vi "Read Field (Variant).vi"(7 "field name":string, 8 "error in (no error)":errorcluster, 9 "type code":T1, 10 "value":variant, 11 "PV Data in":refnum<class "PV Data.lvclass">) -> (0 "error out":errorcluster, 1 "type code out":T1, 2 "value out":variant, 3 "PV Data out":refnum<class "PV Data.lvclass">)   [LabVIEW 2020, in "PV Access.lvlib" / "PV Data.lvlib" / "PV Data.lvclass"]
uses:
  PV Data.lvclass
  PV Data.lvclass/PV Data.ctl
  <vilib>/ErrorRing/Error Ring.xnode
  3e63842f-1b42-44b7-bfbc-53574ae558bd.vi
  0df52538-0c37-4fc1-a2a6-aa64d23bd73e.vi
  ea7cb730-9445-4e63-a674-7488b051f0a2.vi
  ecc6d044-d1d6-4258-b554-93b542f000c4.vi
  f0dd0353-13dc-4229-be36-72f5216b3ba3.vi
  663b7534-5be4-4c26-8693-775dffd107bf.vi
  6d95b702-a3d4-47fa-b99c-6e9c691d9abd.vi
  334379f0-c2c1-4fd4-b37a-a75153a3c3c1.vi
  22215a59-2fe5-468e-8a76-07a567f1422d.vi
  3b673ad6-c2bb-415d-ac32-dac8d0585a62.vi
  4907590c-51dd-452d-854a-3f23d6337043.vi
  91e94b60-106e-4a8f-bb72-5d9817169e6a.vi
  c7390ac7-e1e0-4f30-b90a-9159575d946d.vi
  aaf6655d-cd8e-45f8-b77e-a22837ed21e0.vi
  830d96f2-0dcb-4e12-99cb-9e6dde05f73e.vi
  77dc8c9c-6059-4e17-8748-14fb7ec0ac2f.vi
  a9875d30-4bd9-4a8c-a52c-f68dec12aa6b.vi
  6dbc08b8-92b8-4054-99f1-d97896c52856.vi
  c55a9e90-05cb-4a8a-8098-6274f5663967.vi
  316c9c8d-b543-4ebf-942d-59175514938d.vi
  229b0493-3b28-4ef3-8240-f1556a969e00.vi
  76e9d66a-8186-463b-a0b5-702645c41f9e.vi
  c324c6c0-264f-44f1-9003-e2f03347ce10.vi
  99229403-bf4d-41b1-8e34-2119cf99b534.vi
  60c7cc55-0a77-42d8-819b-5811e97bdf1a.vi
  <vilib>/Utility/error.llb/Error Cluster From Error Code.vi
  Read Field (Boolean Array).vi
  Read Field (Boolean).vi
  Read Field (I8).vi
  Read Field (I8 Array).vi
  Read Field (I16).vi
  Read Field (I32 Array).vi
  Read Field (I32).vi
  Read Field (DBL).vi
  Read Field (DBL Array).vi
  Read Field (I16 Array).vi
  Read Field (I64 Array).vi
  Read Field (I64).vi
  Read Field (SGL Array).vi
  Read Field (SGL).vi
  Read Field (String Array).vi
  Read Field (String).vi
  Read Field (U8 Array).vi
  Read Field (U8).vi
  Read Field (U16 Array).vi
  Read Field (U16).vi
  Read Field (U32 Array).vi
  Read Field (U32).vi
  Read Field (U64 Array).vi
  Read Field (U64).vi
  Type Code.ctl
  PV Data.lvlib
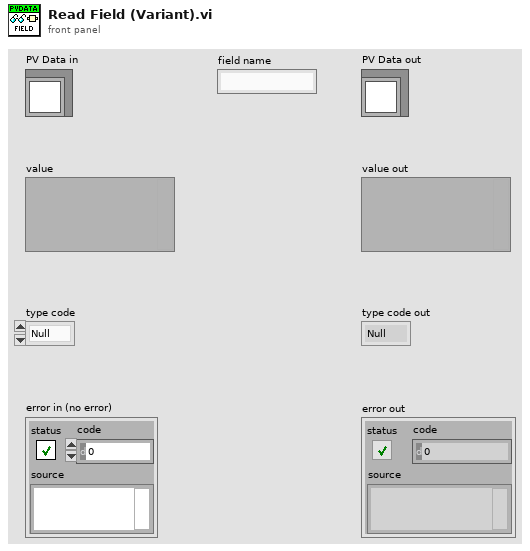
[diagram p1: front panel]
types:
  T1 = typedef "PV Access.lvlib/PV Data.lvlib/Type Code.ctl" = enum8{"Null", "Bool", "BoolA", "Int8", "Int8A", "Int16", "Int16A", "Int32", "Int32A", "Int64", "Int64A", "UInt8", "UInt8A", "UInt16", "UInt16A", "UInt32", "UInt32A", "UInt64", "UInt64A", "Float32", "Float32A", "Float64", "Float64A", "String", "StringA", "Struct", "StructA", "Union", "UnionA", "Any", "AnyA"}
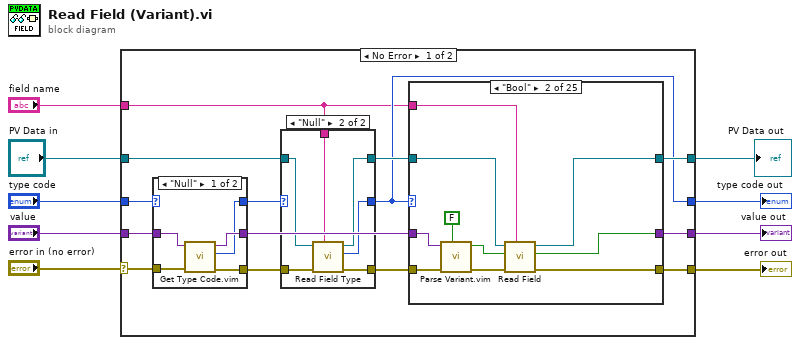
[diagram p0: block diagram]
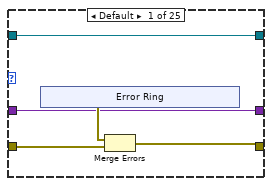
[diagram p4: hidden frame]
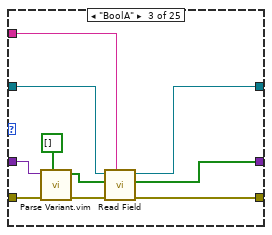
[diagram p5: hidden frame]
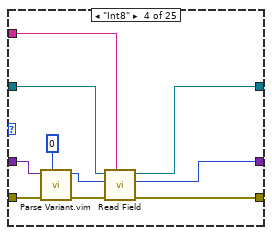
[diagram p6: hidden frame]
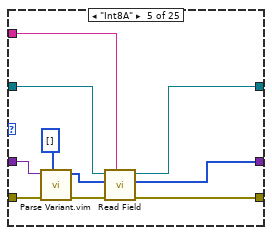
[diagram p7: hidden frame]
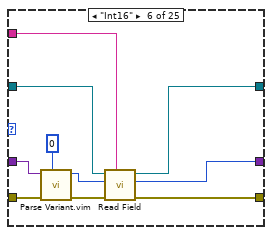
[diagram p8: hidden frame]
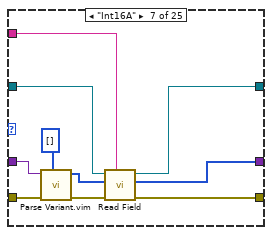
[diagram p9: hidden frame]
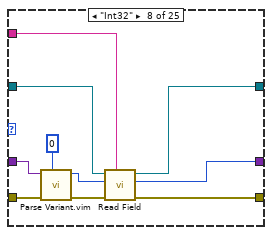
[diagram p10: hidden frame]
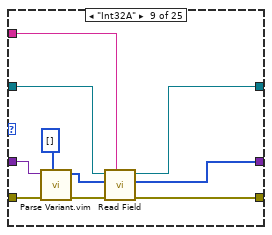
[diagram p11: hidden frame]
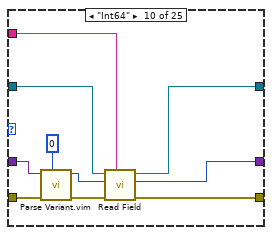
[diagram p12: hidden frame]
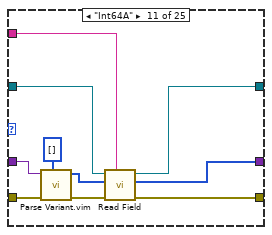
[diagram p13: hidden frame]
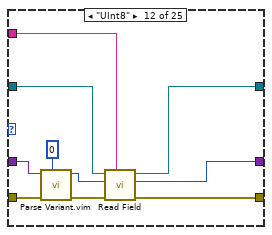
[diagram p14: hidden frame]
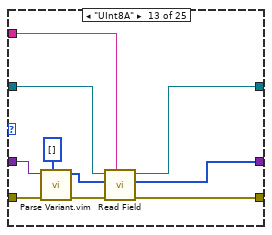
[diagram p15: hidden frame]
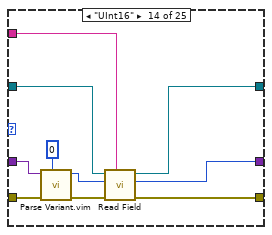
[diagram p16: hidden frame]
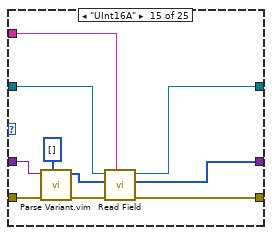
[diagram p17: hidden frame]
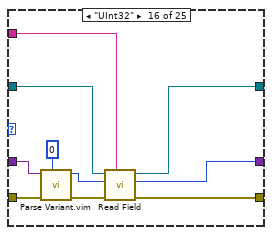
[diagram p18: hidden frame]
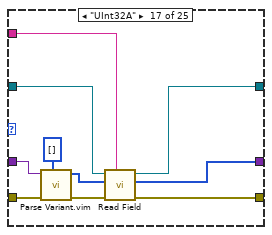
[diagram p19: hidden frame]
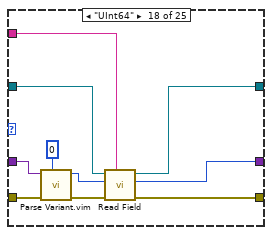
[diagram p20: hidden frame]
diagram:
  n1 = case shown="No Error" "error in (no error)" {
    selector: "error in (no error)" -> [w21 w293]
    tunnel: [w23 w293] -> w8
    tunnel: "PV Data in" -> [w15 w292]
    tunnel: [w22 w292] -> w6
    tunnel: "value" -> [w20 w291]
    tunnel: "type code" -> [w18 w290]
    tunnel: [w12 w291] -> w3
    tunnel: [w11 w290] -> w2
    tunnel: "field name" -> [w10 _]
    frame No Error {
      n2 = case shown="\"Null\"" w18 {
        selector: w18 -> [_ w40]
        tunnel: w21 -> [w37 w39]
        tunnel: [w36 w39] -> w17
        tunnel: w20 -> [w35 w38]
        tunnel: [w34 w38] -> w19
        tunnel: [w33 w40] -> w13
        frame "Null" {
          n3 = call "Get Type Code.vim"("error in"=w37, "value in"=w35) -> ("error out"=w36:errorcluster, "type code"=w33:T1, "value out"=w34:variant)  [unwired: 7 in]
        }
        frame Default {
        }
      }
      n4 = case shown="\"Null\"" w13 {
        selector: w13 -> [w26 _]
        tunnel: w17 -> [w25 w32]
        tunnel: [w25 w31] -> w16
        tunnel: w15 -> [w24 w30]
        tunnel: [w24 w29] -> w14
        tunnel: w10 -> [_ w28]
        tunnel: [w26 w27] -> w11
        frame Default {
        }
        frame "Null" {
          n5 = call "Read Field Type.vi"("field name"=w28, "error in (no error)"=w32, "PV Data in"=w30) -> ("error out"=w31:errorcluster, "type code"=w27:T1, "PV Data out"=w29:refnum<class "PV Data.lvclass">)  [unwired: 6 in]
        }
      }
      n6 = case shown="\"Bool\"" w11 {
        tunnel: [w44 w56 w67 w77 w87 w97 w107 w117 w127 w137 w148 w157 w167 w177 w187 w197 w207 w217 w227 w237 w247 w257 w267 w277 w287] -> w23
        tunnel: w16 -> [w45 w59 w69 w79 w89 w99 w109 w119 w129 w139 w149 w159 w169 w179 w189 w199 w209 w219 w229 w239 w249 w259 w269 w279 w289]
        tunnel: [w42 w54 w65 w76 w85 w95 w105 w115 w125 w135 w146 w155 w165 w176 w185 w195 w206 w215 w225 w235 w245 w255 w265 w275 w285] -> w22
        tunnel: [w41 w53 w63 w74 w83 w93 w103 w113 w123 w133 w144 w153 w163 w174 w183 w193 w204 w213 w223 w233 w243 w253 w263 w273 w283] -> w12
        tunnel: w14 -> [w42 w52 w62 w73 w82 w92 w102 w112 w122 w132 w142 w152 w162 w173 w182 w192 w203 w212 w222 w232 w242 w252 w262 w272 w282]
        tunnel: w19 -> [w41 w51 w60 w70 w80 w90 w100 w110 w120 w130 w140 w150 w160 w170 w180 w190 w200 w210 w220 w230 w240 w250 w260 w270 w280]
        tunnel: w10 -> [_ w50 w61 w71 w81 w91 w101 w111 w121 w131 w141 w151 w161 w171 w181 w191 w201 w211 w221 w231 w241 w251 w261 w271 w281]
        frame Default {
          n7 = xnode "Error Ring"() -> ("error out"=w43:errorcluster)
          n8 = Merge Errors(w43, w45) -> (w44:errorcluster)
        }
        frame "Bool" {
          n9 = call "Parse Variant.vim"("default"=FALSE, "error in (no error)"=w59, "value"=w51) -> ("error out"=w57:errorcluster, "value out"=w55:bool)  [unwired: 7 in]
          n10 = call-poly "Read Field.vi"("field name"=w50, "error in (no error)"=w57, "default"=w55, "PV Data in"=w52) -> ("error out"=w56:errorcluster, "value"=w53:bool, "PV Data out"=w54:refnum<class "PV Data.lvclass">)  [unwired: 5 in]
        }
        frame "BoolA" {
          n11 = call "Parse Variant.vim"("default"=bool[] [], "error in (no error)"=w69, "value"=w60) -> ("error out"=w68:errorcluster, "value out"=w66:bool[])  [unwired: 7 in]
          n12 = call-poly "Read Field.vi"("field name"=w61, "error in (no error)"=w68, "default"=w66, "PV Data in"=w62) -> ("error out"=w67:errorcluster, "value"=w63:bool[], "PV Data out"=w65:refnum<class "PV Data.lvclass">)  [unwired: 5 in]
        }
        frame "Int8" {
          n13 = call "Parse Variant.vim"("default"=i8 0, "error in (no error)"=w79, "value"=w70) -> ("error out"=w78:errorcluster, "value out"=w72:i8)  [unwired: 7 in]
          n14 = call-poly "Read Field.vi"("field name"=w71, "error in (no error)"=w78, "default"=w72, "PV Data in"=w73) -> ("error out"=w77:errorcluster, "value"=w74:i8, "PV Data out"=w76:refnum<class "PV Data.lvclass">)  [unwired: 5 in]
        }
        frame "Int8A" {
          n15 = call "Parse Variant.vim"("default"=i8[] [], "error in (no error)"=w89, "value"=w80) -> ("error out"=w88:errorcluster, "value out"=w86:i8[])  [unwired: 7 in]
          n16 = call-poly "Read Field.vi"("field name"=w81, "error in (no error)"=w88, "default"=w86, "PV Data in"=w82) -> ("error out"=w87:errorcluster, "value"=w83:i8[], "PV Data out"=w85:refnum<class "PV Data.lvclass">)  [unwired: 5 in]
        }
        frame "Int16" {
          n17 = call "Parse Variant.vim"("default"=i16 0, "error in (no error)"=w99, "value"=w90) -> ("error out"=w98:errorcluster, "value out"=w96:i16)  [unwired: 7 in]
          n18 = call-poly "Read Field.vi"("field name"=w91, "error in (no error)"=w98, "default"=w96, "PV Data in"=w92) -> ("error out"=w97:errorcluster, "value"=w93:i16, "PV Data out"=w95:refnum<class "PV Data.lvclass">)  [unwired: 5 in]
        }
        frame "Int16A" {
          n19 = call "Parse Variant.vim"("default"=i16[] [], "error in (no error)"=w109, "value"=w100) -> ("error out"=w108:errorcluster, "value out"=w106:i16[])  [unwired: 7 in]
          n20 = call-poly "Read Field.vi"("field name"=w101, "error in (no error)"=w108, "default"=w106, "PV Data in"=w102) -> ("error out"=w107:errorcluster, "value"=w103:i16[], "PV Data out"=w105:refnum<class "PV Data.lvclass">)  [unwired: 5 in]
        }
        frame "Int32" {
          n21 = call "Parse Variant.vim"("default"=0, "error in (no error)"=w119, "value"=w110) -> ("error out"=w118:errorcluster, "value out"=w116:i32)  [unwired: 7 in]
          n22 = call-poly "Read Field.vi"("field name"=w111, "error in (no error)"=w118, "default"=w116, "PV Data in"=w112) -> ("error out"=w117:errorcluster, "value"=w113:i32, "PV Data out"=w115:refnum<class "PV Data.lvclass">)  [unwired: 5 in]
        }
        frame "Int32A" {
          n23 = call "Parse Variant.vim"("default"=i32[] [], "error in (no error)"=w129, "value"=w120) -> ("error out"=w128:errorcluster, "value out"=w126:i32[])  [unwired: 7 in]
          n24 = call-poly "Read Field.vi"("field name"=w121, "error in (no error)"=w128, "default"=w126, "PV Data in"=w122) -> ("error out"=w127:errorcluster, "value"=w123:i32[], "PV Data out"=w125:refnum<class "PV Data.lvclass">)  [unwired: 5 in]
        }
        frame "Int64" {
          n25 = call "Parse Variant.vim"("default"=i64 0, "error in (no error)"=w139, "value"=w130) -> ("error out"=w138:errorcluster, "value out"=w136:i64)  [unwired: 7 in]
          n26 = call-poly "Read Field.vi"("field name"=w131, "error in (no error)"=w138, "default"=w136, "PV Data in"=w132) -> ("error out"=w137:errorcluster, "value"=w133:i64, "PV Data out"=w135:refnum<class "PV Data.lvclass">)  [unwired: 5 in]
        }
        frame "Int64A" {
          n27 = call "Parse Variant.vim"("default"=i64[] [], "error in (no error)"=w149, "value"=w140) -> ("error out"=w143:errorcluster, "value out"=w147:i64[])  [unwired: 7 in]
          n28 = call-poly "Read Field.vi"("field name"=w141, "error in (no error)"=w143, "default"=w147, "PV Data in"=w142) -> ("error out"=w148:errorcluster, "value"=w144:i64[], "PV Data out"=w146:refnum<class "PV Data.lvclass">)  [unwired: 5 in]
        }
        frame "UInt8" {
          n29 = call "Parse Variant.vim"("default"=u8 0, "error in (no error)"=w159, "value"=w150) -> ("error out"=w158:errorcluster, "value out"=w156:u8)  [unwired: 7 in]
          n30 = call-poly "Read Field.vi"("field name"=w151, "error in (no error)"=w158, "default"=w156, "PV Data in"=w152) -> ("error out"=w157:errorcluster, "value"=w153:u8, "PV Data out"=w155:refnum<class "PV Data.lvclass">)  [unwired: 5 in]
        }
        frame "UInt8A" {
          n31 = call "Parse Variant.vim"("default"=u8[] [], "error in (no error)"=w169, "value"=w160) -> ("error out"=w168:errorcluster, "value out"=w166:u8[])  [unwired: 7 in]
          n32 = call-poly "Read Field.vi"("field name"=w161, "error in (no error)"=w168, "default"=w166, "PV Data in"=w162) -> ("error out"=w167:errorcluster, "value"=w163:u8[], "PV Data out"=w165:refnum<class "PV Data.lvclass">)  [unwired: 5 in]
        }
        frame "UInt16" {
          n33 = call "Parse Variant.vim"("default"=u16 0, "error in (no error)"=w179, "value"=w170) -> ("error out"=w178:errorcluster, "value out"=w172:u16)  [unwired: 7 in]
          n34 = call-poly "Read Field.vi"("field name"=w171, "error in (no error)"=w178, "default"=w172, "PV Data in"=w173) -> ("error out"=w177:errorcluster, "value"=w174:u16, "PV Data out"=w176:refnum<class "PV Data.lvclass">)  [unwired: 5 in]
        }
        frame "UInt16A" {
          n35 = call "Parse Variant.vim"("default"=u16[] [], "error in (no error)"=w189, "value"=w180) -> ("error out"=w188:errorcluster, "value out"=w186:u16[])  [unwired: 7 in]
          n36 = call-poly "Read Field.vi"("field name"=w181, "error in (no error)"=w188, "default"=w186, "PV Data in"=w182) -> ("error out"=w187:errorcluster, "value"=w183:u16[], "PV Data out"=w185:refnum<class "PV Data.lvclass">)  [unwired: 5 in]
        }
        frame "UInt32" {
          n37 = call "Parse Variant.vim"("default"=u32 0, "error in (no error)"=w199, "value"=w190) -> ("error out"=w198:errorcluster, "value out"=w196:u32)  [unwired: 7 in]
          n38 = call-poly "Read Field.vi"("field name"=w191, "error in (no error)"=w198, "default"=w196, "PV Data in"=w192) -> ("error out"=w197:errorcluster, "value"=w193:u32, "PV Data out"=w195:refnum<class "PV Data.lvclass">)  [unwired: 5 in]
        }
        frame "UInt32A" {
          n39 = call "Parse Variant.vim"("default"=u32[] [], "error in (no error)"=w209, "value"=w200) -> ("error out"=w208:errorcluster, "value out"=w202:u32[])  [unwired: 7 in]
          n40 = call-poly "Read Field.vi"("field name"=w201, "error in (no error)"=w208, "default"=w202, "PV Data in"=w203) -> ("error out"=w207:errorcluster, "value"=w204:u32[], "PV Data out"=w206:refnum<class "PV Data.lvclass">)  [unwired: 5 in]
        }
        frame "UInt64" {
          n41 = call "Parse Variant.vim"("default"=u64 0, "error in (no error)"=w219, "value"=w210) -> ("error out"=w218:errorcluster, "value out"=w216:u64)  [unwired: 7 in]
          n42 = call-poly "Read Field.vi"("field name"=w211, "error in (no error)"=w218, "default"=w216, "PV Data in"=w212) -> ("error out"=w217:errorcluster, "value"=w213:u64, "PV Data out"=w215:refnum<class "PV Data.lvclass">)  [unwired: 5 in]
        }
        frame "UInt64A" {
          n43 = call "Parse Variant.vim"("default"=u64[] [], "error in (no error)"=w229, "value"=w220) -> ("error out"=w228:errorcluster, "value out"=w226:u64[])  [unwired: 7 in]
          n44 = call-poly "Read Field.vi"("field name"=w221, "error in (no error)"=w228, "default"=w226, "PV Data in"=w222) -> ("error out"=w227:errorcluster, "value"=w223:u64[], "PV Data out"=w225:refnum<class "PV Data.lvclass">)  [unwired: 5 in]
        }
        frame "Float32" {
          n45 = call "Parse Variant.vim"("default"=sgl 0.0, "error in (no error)"=w239, "value"=w230) -> ("error out"=w238:errorcluster, "value out"=w236:sgl)  [unwired: 7 in]
          n46 = call-poly "Read Field.vi"("field name"=w231, "error in (no error)"=w238, "default"=w236, "PV Data in"=w232) -> ("error out"=w237:errorcluster, "value"=w233:sgl, "PV Data out"=w235:refnum<class "PV Data.lvclass">)  [unwired: 5 in]
        }
        frame "Float64" {
          n47 = call "Parse Variant.vim"("default"=0.0, "error in (no error)"=w249, "value"=w240) -> ("error out"=w248:errorcluster, "value out"=w246:dbl)  [unwired: 7 in]
          n48 = call-poly "Read Field.vi"("field name"=w241, "error in (no error)"=w248, "default"=w246, "PV Data in"=w242) -> ("error out"=w247:errorcluster, "value"=w243:dbl, "PV Data out"=w245:refnum<class "PV Data.lvclass">)  [unwired: 5 in]
        }
        frame "Float32A" {
          n49 = call "Parse Variant.vim"("default"=sgl[] [], "error in (no error)"=w259, "value"=w250) -> ("error out"=w258:errorcluster, "value out"=w256:sgl[])  [unwired: 7 in]
          n50 = call-poly "Read Field.vi"("field name"=w251, "error in (no error)"=w258, "default"=w256, "PV Data in"=w252) -> ("error out"=w257:errorcluster, "value"=w253:sgl[], "PV Data out"=w255:refnum<class "PV Data.lvclass">)  [unwired: 5 in]
        }
        frame "Float64A" {
          n51 = call "Parse Variant.vim"("default"=dbl[] [], "error in (no error)"=w269, "value"=w260) -> ("error out"=w268:errorcluster, "value out"=w266:dbl[])  [unwired: 7 in]
          n52 = call-poly "Read Field.vi"("field name"=w261, "error in (no error)"=w268, "default"=w266, "PV Data in"=w262) -> ("error out"=w267:errorcluster, "value"=w263:dbl[], "PV Data out"=w265:refnum<class "PV Data.lvclass">)  [unwired: 5 in]
        }
        frame "String" {
          n53 = call "Parse Variant.vim"("default"="", "error in (no error)"=w279, "value"=w270) -> ("error out"=w278:errorcluster, "value out"=w276:string)  [unwired: 7 in]
          n54 = call-poly "Read Field.vi"("field name"=w271, "error in (no error)"=w278, "default"=w276, "PV Data in"=w272) -> ("error out"=w277:errorcluster, "value"=w273:string, "PV Data out"=w275:refnum<class "PV Data.lvclass">)  [unwired: 5 in]
        }
        frame "StringA" {
          n55 = call "Parse Variant.vim"("default"=string[] [], "error in (no error)"=w289, "value"=w280) -> ("error out"=w288:errorcluster, "value out"=w286:string[])  [unwired: 7 in]
          n56 = call-poly "Read Field.vi"("field name"=w281, "error in (no error)"=w288, "default"=w286, "PV Data in"=w282) -> ("error out"=w287:errorcluster, "value"=w283:string[], "PV Data out"=w285:refnum<class "PV Data.lvclass">)  [unwired: 5 in]
        }
      }
    }
    frame Error {
    }
  }
  "value out" <- w3
  "error out" <- w8
  "PV Data out" <- w6
  "type code out" <- w2
